vi "test20-LosslessRegisterStateMultipleTimes.vi"(8 "error in (no error)":errorcluster, 11 "TestCase in":refnum<class "testcase-CSMBroadcast.lvclass">) -> (0 "error out":errorcluster, 3 "TestCase out":refnum<class "testcase-CSMBroadcast.lvclass">)   [LabVIEW 2017, in "testcase-CSMBroadcast.lvclass"]
uses:
  testcase-CSMBroadcast.lvclass
  bc269a46-fbd8-4fbd-ac76-06990d02385a.vi
  8d37a2f4-20d8-4102-818c-5a8acec6f80e.vi
  src/user.lib/_NEVSTOP/Communicable State Machine(CSM)/AdvanceAPI/CSM - Get Module Attribute.vi
  <vilib>/addons/_JKI Toolkits/VI Tester/TestCase.llb/TestCase.lvclass
  src/user.lib/_NEVSTOP/Communicable State Machine(CSM)/Communicable State Machine.lvlib
  CSM/CSM-Testcase.lvlib
  C:/Program Files (x86)/National Instruments/LabVIEW 2017/vi.lib/addons/_JKI Toolkits/VI Tester/TestCase.llb/TestCase.lvclass
panel:
  out "LoopCount":i32
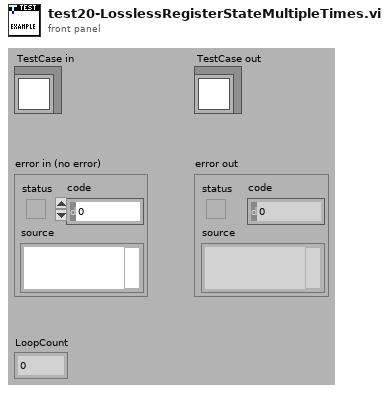
[diagram p1: front panel]
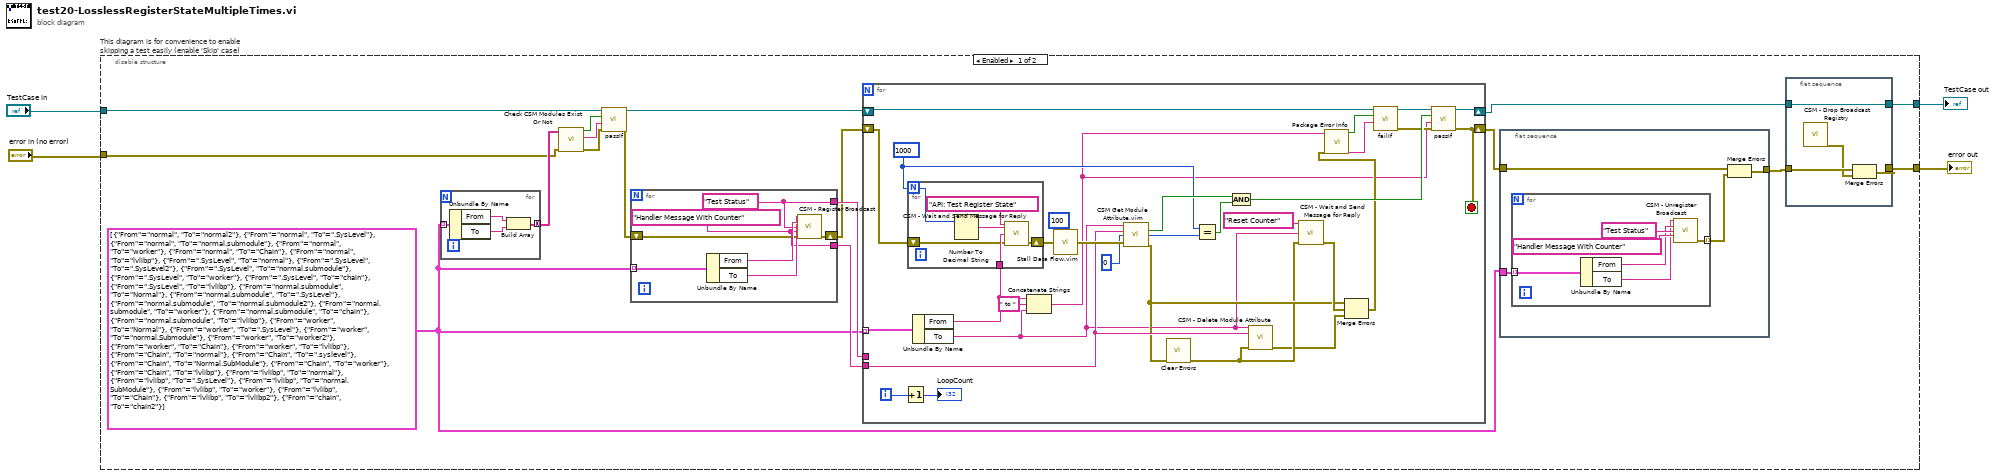
[diagram p0: block diagram]
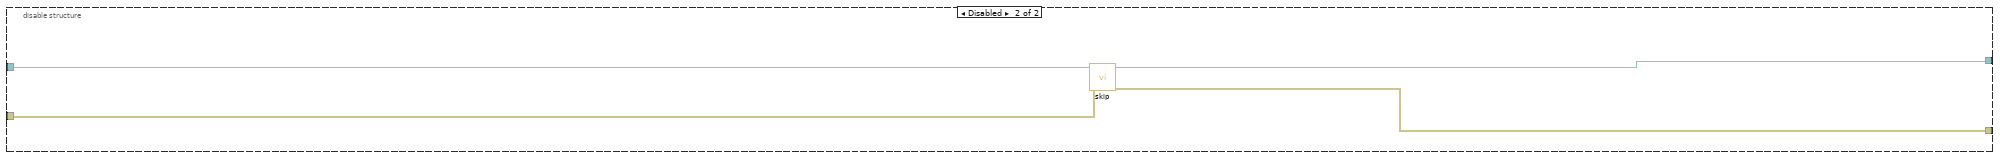
[diagram p2: hidden frame]
diagram:
  n1 = disable-structure "This diagram is for convenience to enable skipping a test easily (enable 'Skip' case)" shown="Enabled" {
    disable-tunnel: "TestCase in" -> [w10 w87]
    disable-tunnel: [w16 w85] -> w2
    disable-tunnel: [w19 w86] -> w1
    disable-tunnel: "error in (no error)" -> [w7 w84]
    frame Enabled {
      w8 = cluster{"From":string, "To":string}[] [{"From"="normal", "To"="normal2"}, {"From"="normal", "To"=".SysLevel"}, {"From"="normal", "To"="normal.submodule"}, {"From"="normal", "To"="worker"}, {"From"="normal", "To"="Chain"}, {"From"="normal", "To"="lvlibp"}, {"From"=".SysLevel", "To"="normal"}, {"From"=".SysLevel", "To"=".SysLevel2"}, {"From"=".SysLevel", "To"="normal.submodule"}, {"From"=".SysLevel", "To"="worker"}, {"From"=".SysLevel", "To"="chain"}, {"From"=".SysLevel", "To"="lvlibp"}, {"From"="normal.submodule", "To"="Normal"}, {"From"="normal.submodule", "To"=".SysLevel"}, {"From"="normal.submodule", "To"="normal.submodule2"}, {"From"="normal.submodule", "To"="worker"}, {"From"="normal.submodule", "To"="chain"}, {"From"="normal.submodule", "To"="lvlibp"}, {"From"="worker", "To"="Normal"}, {"From"="worker", "To"=".SysLevel"}, {"From"="worker", "To"="normal.Submodule"}, {"From"="worker", "To"="worker2"}, {"From"="worker", "To"="Chain"}, {"From"="worker", "To"="lvlibp"}, {"From"="Chain", "To"="normal"}, {"From"="Chain", "To"=".syslevel"}, {"From"="Chain", "To"="Normal.SubModule"}, {"From"="Chain", "To"="worker"}, {"From"="Chain", "To"="lvlibp"}, {"From"="lvlibp", "To"="normal"}, {"From"="lvlibp", "To"=".SysLevel"}, {"From"="lvlibp", "To"="normal.SubModule"}, {"From"="lvlibp", "To"="worker"}, {"From"="lvlibp", "To"="Chain"}, {"From"="lvlibp", "To"="lvlibp2"}, {"From"="chain", "To"="chain2"}]
      n2 = for {
        tunnel: w8 -> [w25] mode=indexing
        tunnel: [w22] -> w13 mode=concatenating
        n3 = Unbundle By Name(w25) -> ("From"=w24:string, "To"=w23:string)
        n4 = Build Array(w24, w23) -> (w22:string[])
      }
      n5 = call "Check CSM Modules Exist Or Not.vi"("error in"=w7, "CSM names in"=w13) -> ("error out"=w11:errorcluster, "Debug string"=w12:string, "All Modules Exist?"=w14:bool)  [unwired: 7 in]
      n6 = call-dynamic "passIf.vi"("error in (no error)"=w11, "message (\"\")"=w12, "pass"=w14, "TestCase in"=w10) -> ("error out"=w6:errorcluster, "TestCase out"=w9:refnum<class "testcase-CSMBroadcast.lvclass">)  [unwired: 6 in]
      n7 = for {
        tunnel: w8 -> [w42] mode=indexing
        tunnel: [w38] -> w18
        tunnel: [w37] -> w15
        shift-right: [w39] -> w5
        shift-left: w6 -> [w36]
        w37 = "Handler Message With Counter" ("Response Message (If \"\", Same as Source Message)")
        w38 = "Test Status" ("Status")
        n8 = Unbundle By Name(w42) -> ("From"=w41:string, "To"=w40:string)
        n9 = call "CSM - Register Broadcast.vi"("CSM Name(Empty for Broadcast Event)"=w40, "Source CSM Name (* as Default)"=w41, "Trigger"=w38, "API (If \"\", Same as Trigger)"=w37, "Error In"=w36) -> ("error out"=w39:errorcluster)  [unwired: 9 in, 1 out]
      }
      n10 = for {
        tunnel: w8 -> [w77] mode=indexing
        shift-right: [w72] -> w17
        shift-left: w9 -> [w54]
        shift-right: [w70] -> w21
        shift-left: w5 -> [w57]
        tunnel: w18 -> [_]
        tunnel: w15 -> [w69]
        i -> [w68]
        stop <- w70 stop-if-true
        w64 = 1000
        n11 = Increment(x=w68) -> (x+1=→"LoopCount":i32)
        n12 = Unbundle By Name(w77) -> ("From"=w50:string, "To"=w49:string)
        n13 = for {
          N: w64 -> [w78]
          tunnel: w50 -> [w81]
          shift-right: [w82] -> w76
          shift-left: w57 -> [w80]
          n14 = Number To Decimal String(number=w78) -> (decimal integer string=w79:string)  [unwired: 1 in]
          n15 = call "CSM - Wait and Send Message for Reply.vi"("State"="API: Test Register State", "Arguments (\"\")"=w79, "Target Module"=w81, "Error In (No Error)"=w80) -> ("error out"=w82:errorcluster)  [unwired: 8 in, 3 out]
        }
        n16 = Concatenate Strings(w50, " to " ("string"), w49) -> (w47:string)
        n17 = call "Stall Data Flow.vim"("value in"=w76, "milliseconds to wait"=u32 100) -> ("value out"=w74:errorcluster)  [unwired: 1 out]
        n18 = call "CSM Get Module Attribute.vim"("CSM Name"=w49, "Attribute"=w69, "Default Value (Empty Variant)"=u32 0, "Error In"=w74) -> ("Found"=w73:bool, "Value"=w65:u32, "error out"=w60:errorcluster)  [unwired: 7 in, 2 out]
        n19 = call <vilib>:"Clear Errors.vi"("error in (no error)"=w60) -> ("error out"=w59:errorcluster)  [unwired: 5 in, 1 out]
        n20 = Equal?(x=w64, y=w65) -> (x = y?=w63:bool)
        n21 = Compound Arithmetic op=AND(w73, w63) -> (w71:bool)
        n22 = call "CSM - Delete Module Attribute.vi"("CSM Name"=w49, "Attribute"=w69, "Error In"=w59) -> ("error out"=w58:errorcluster)  [unwired: 9 in, 3 out]
        n23 = call "CSM - Wait and Send Message for Reply.vi"("State"="Reset Counter", "Target Module"=w49, "Error In (No Error)"=w59) -> ("error out"=w61:errorcluster)  [unwired: 9 in, 3 out]
        n24 = Merge Errors(w60, w61, w58) -> (w51:errorcluster)
        n25 = call "Package Error Info.vi"("error in"=w51, "String in"=w47) -> ("packed error info out"=w55:string, "error status"=w56:bool)  [unwired: 8 in]
        n26 = call-dynamic "failIf.vi"("message (\"\")"=w55, "fail"=w56, "TestCase in"=w54) -> ("error out"=w52:errorcluster, "TestCase out"=w53:refnum<class "testcase-CSMBroadcast.lvclass">)  [unwired: 7 in]
        n27 = call-dynamic "passIf.vi"("error in (no error)"=w52, "message (\"\")"=w47, "pass"=w71, "TestCase in"=w53) -> ("error out"=w70:errorcluster, "TestCase out"=w72:refnum<class "testcase-CSMBroadcast.lvclass">)  [unwired: 6 in]
      }
      n28 = flat-sequence {
        tunnel: w8 -> [w26]
        tunnel: w21 -> [w29]
        tunnel: [w28] -> w20
        frame #0 {
          n29 = for {
            tunnel: w26 -> [w30] mode=indexing
            tunnel: [w31] -> w27 mode=indexing
            n30 = Unbundle By Name(w30) -> ("From"=w33:string, "To"=w32:string)
            n31 = call "CSM - Unregister Broadcast.vi"("CSM Name(Empty for Broadcast Event)"=w32, "Source CSM Name (* as Default)"=w33, "Trigger"="Test Status" ("Status"), "API (\"*\" as Default)"="Handler Message With Counter" ("Response Message (If \"\", Same as Source Message)")) -> ("error out"=w31:errorcluster)  [unwired: 10 in, 1 out]
          }
          n32 = Merge Errors(w29, w27) -> (w28:errorcluster)
        }
      }
      n33 = flat-sequence {
        tunnel: w20 -> [w46]
        tunnel: [w45] -> w19
        tunnel: [w44] -> w16
        tunnel: w17 -> [w44]
        frame #0 {
          n34 = call "CSM - Drop Broadcast Registry.vi"() -> ("error out"=w43:errorcluster)  [unwired: 15 in]
          n35 = Merge Errors(w46, w43) -> (w45:errorcluster)
        }
      }
    }
    frame Disabled {
      # "skip test result while test is under development"
      n36 = call <vilib>:"skip.vi"("error in (no error)"=w84, "TestCase in"=w87) -> ("error out"=w86:errorcluster, "TestCase out"=w85:refnum<class "testcase-CSMBroadcast.lvclass">)  [unwired: 8 in]
    }
  }
  "error out" <- w1
  "TestCase out" <- w2
